vi "FFT-THD.vi"(11 "TF Corr IMon FFT":T1={"f0"=0.0, "df"=15.873015873016348, "magnitude"=array[31500 elements], "phase"=array[31500 elements], "PSD"=array[31500 elements]}) -> (3 "THD":dbl)   [LabVIEW 2021]
uses:
  MPS_Labview/MPS_global_variables.vi
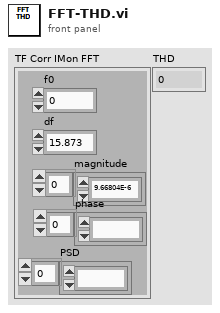
[diagram p1: front panel]
types:
  T1 = cluster{"f0":dbl, "df":dbl, "magnitude":dbl[], "phase":dbl[], "PSD":dbl[]}
  T2 = cluster{"sample rate":dbl, "Transmit frequency":dbl, "Transmit amplitude":dbl, "sample rate digital out":dbl, "TX cycles":i32, "sample rate DAQ1":dbl, "Receive frequency":dbl, "Receive range":dbl, "TX harmonics":dbl[]}
  T3 = cluster{"sample rate":dbl, "Tx freq":dbl, "Tx amp":dbl, "Tx cycles\nSpectroscopy":dbl, "Bias amp":dbl, "Bias freq":dbl, "Receive range":dbl, "Bias Periods\nMagnetometry":dbl, "Tx Freq Division Factor":dbl, "Drive Periods per Bias":dbl, "TX harmonics":dbl[]}
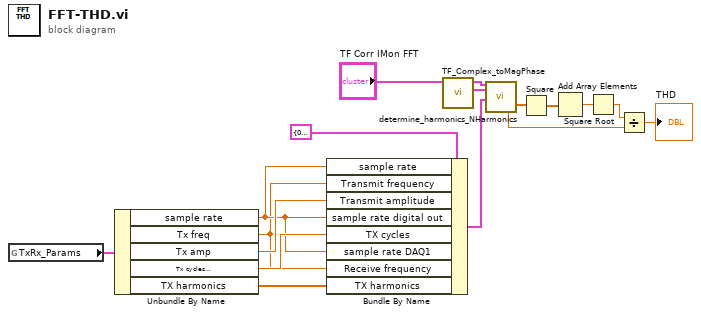
[diagram p0: block diagram]
diagram:
  n1 = global read "MPS_global_variables.vi" "TxRx_Params"() -> (w12:T3)
  n2 = Unbundle By Name(w12) -> ("sample rate"=w9:dbl, "Tx freq"=w8:dbl, "Tx amp"=w11:dbl, "Tx cycles\nSpectroscopy"=w10:dbl, "TX harmonics"=w7:dbl[])
  n3 = Bundle By Name(cluster=T2 {"sample rate"=0.0, "Transmit frequency"=0.0, "Transmit amplitude"=0.0, "sample rate digital out"=0.0, "TX cycles"=0, "sample rate DAQ1"=0.0, "Receive frequency"=0.0, "Receive range"=0.0, "TX harmonics"=[]} ("TxRxParams"), "sample rate"=w9, "Transmit frequency"=w8, "Transmit amplitude"=w11, "sample rate digital out"=w9, "TX cycles"=w10, "sample rate DAQ1"=w9, "Receive frequency"=w8, "TX harmonics"=w7) -> (w13:T2)
  n4 = call "TF_Complex_toMagPhase.vi"("TF Corr Rx FFT Mag"="TF Corr IMon FFT") -> ("TF Phase"=w15:cluster{"f0":dbl, "df":dbl, "magnitude":dbl[]}, "TF Mag"=w16:cluster{"f0":dbl, "df":dbl, "magnitude":dbl[]})  [unwired: 4 in, 5 out]
  n5 = call "determine_harmonics_NHarmonics.vi"("FFT magnitude"=w16, "FFT phase"=w15, "TxRxParams"=w13) -> ("f0 mag"=w6:dbl, "mag 2f0-Nf0"=w5:dbl[])  [unwired: 11 in, 4 out]
  n6 = Square(x=w5) -> (x^2=w4:dbl[])
  n7 = Add Array Elements(numeric array=w4) -> (sum=w3:dbl)
  n8 = Square Root(x=w3) -> (sqrt(x)=w2:dbl)
  n9 = Divide(x=w2, y=w6) -> (x/y=→"THD":dbl)
